vi "Initialize Version.vi"(8 "error in (no error)":errorcluster, 11 "Core Transfers Configuration in":refnum<class "Core Transfers Configuration.lvclass">) -> (0 "error out":errorcluster, 3 "Core Transfers Configuration out":refnum<class "Core Transfers Configuration.lvclass">)   [LabVIEW 2017, in "DSF Core.lvlib" / "Core Transfers Configuration.lvclass"]
uses:
  Core Transfers Configuration.lvclass
  Typedefs/DSF Version Info.ctl
  DSF Core.lvlib
  C:/Git/DSF/Core/Classes/Configuration/Configuration.lvclass
  Configuration.lvclass
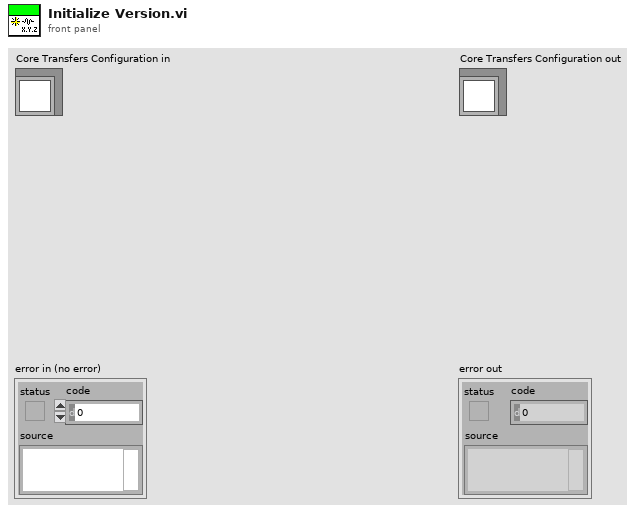
[diagram p1: front panel]
types:
  T1 = typedef "DSF Core.lvlib/DSF Version Info.ctl" = cluster{"major":u32, "minor":u32, "fix":u32, "build":string}
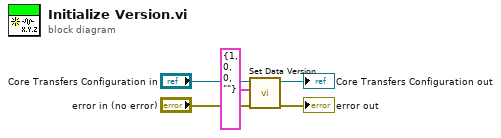
[diagram p0: block diagram]
diagram:
  n1 = call "Set Data Version.vi"("error in (no error)"="error in (no error)", "data version"=T1 {"major"=1, "minor"=0, "fix"=0, "build"=""} ("format version"), "Configuration in"="Core Transfers Configuration in") -> ("error out"=→"error out":errorcluster, "Configuration out"=→"Core Transfers Configuration out":refnum<class "Configuration.lvclass">)  [unwired: 7 in]
